vi "_Enabled or value string.vi"(3 "Initial String":string, 4 "Enabled or Value":i32(ring) items=["Off", "On", "Value"], 5 "Value":dbl) -> (2 "Resulting String":string)   [LabVIEW 2020, in "Rohde&Schwarz CMWXP NR FR1 Measurement.lvlib"]
uses:
  <instrlib>/Rohde&Schwarz CMWXP NR FR1 Measurement/Rohde&Schwarz CMWXP NR FR1 Measurement.lvlib
  <instrlib>/Rohde&Schwarz CMWXP NR FR1 Measurement/Private/rsidr_core.llb/rsidr_core.lvlib
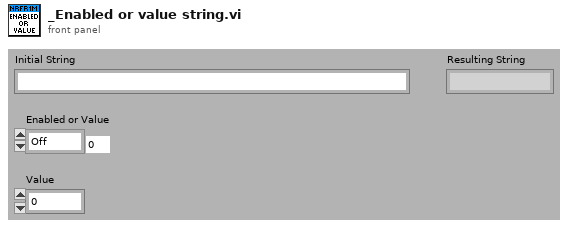
[diagram p1: front panel]
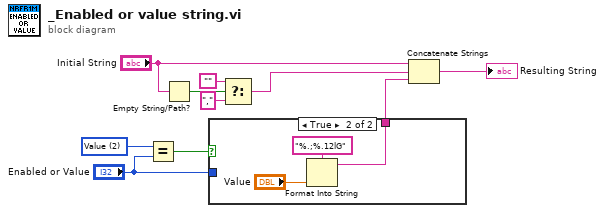
[diagram p0: block diagram]
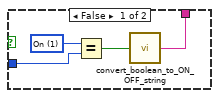
[diagram p2: hidden frame]
diagram:
  w5 = 2 items=["Off", "On", "Value"] ("Enabled or Value")
  n1 = Equal?(x=w5, y="Enabled or Value") -> (x = y?=w4:bool)
  n2 = Empty String/Path?(string/path="Initial String") -> (empty?=w9:bool)
  n3 = case shown="True" w4 {
    tunnel: "Enabled or Value" -> [w13 _]
    tunnel: [w11 w15] -> w2
    frame False {
      w14 = 1 items=["Off", "On", "Value"] ("Enabled or Value")
      n4 = Equal?(x=w14, y=w13) -> (x = y?=w12:bool)
      n5 = call <instrlib>:"convert_boolean_to_ON_OFF_string.vi"("boolean value in"=w12) -> ("string value out"=w11:string)  [unwired: 4 in]
    }
    frame True {
      n6 = Format Into String(format string="%.;%.12lG", "Value") -> (resulting string=w15:string)  [unwired: 2 in, 1 out]
    }
  }
  n7 = Select(t="", s=w9, f=",") -> (s? t:f=w6:string)
  n8 = Concatenate Strings("Initial String", w6, w2) -> (→"Resulting String":string)
